vi "~sequence tester.vi"() -> ()   [LabVIEW 2017]
uses:
  Classes/Sequence/SequenceSubvis/TestStep.ctl
  Classes/Sequence/SequenceSubvis/RF Direction.ctl
  Classes/Sequence/SequenceSubvis/PolarizationSelect.ctl
  StepCmdProperties.ctl
  NewTestProperties.ctl
panel:
  out "New Setups":T1[](array[typedef])
  out "Array":T3[](array[typedef])
  in  "Sequence":T4[](array[typedef])
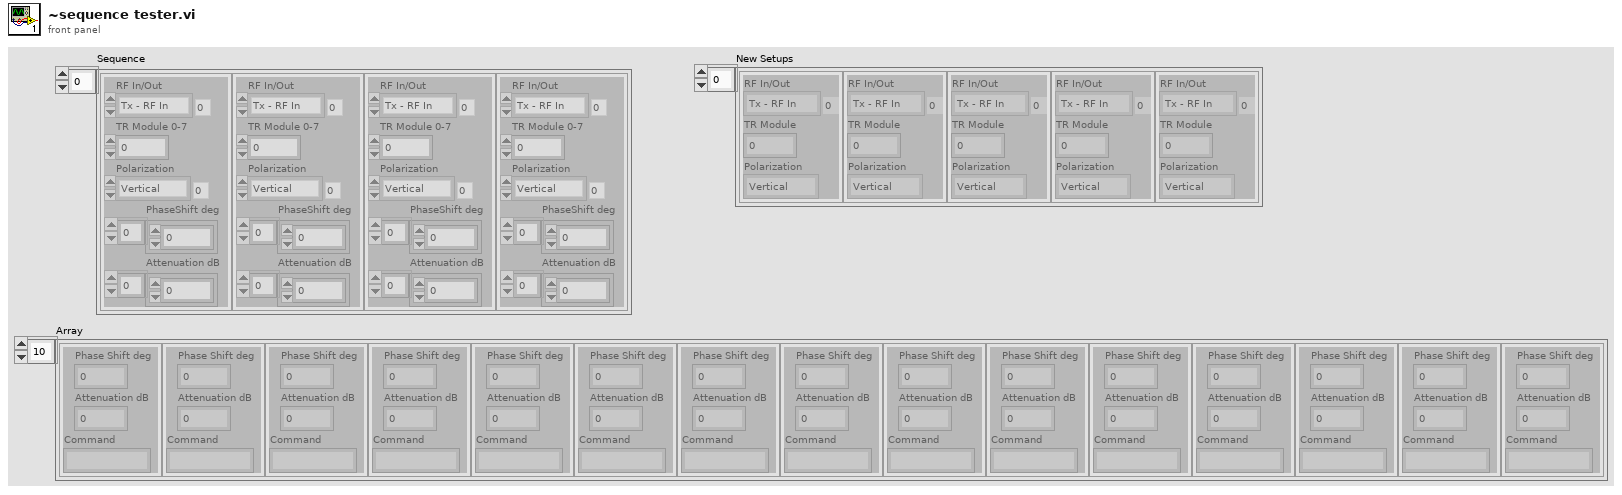
[diagram p1: front panel]
types:
  T1 = typedef "NewTestProperties.ctl" = cluster{"RF In/Out":T2, "TR Module":i32, "Polarization":enum16{"Vertical", "Horizontal"}}
  T2 = typedef "RF Direction.ctl" = enum16{"Tx - RF In", "Rx - RF Out"}
  T3 = typedef "StepCmdProperties.ctl" = cluster{"Phase Shift deg":dbl, "Attenuation dB":dbl, "Command":string}
  T4 = typedef "TestStep.ctl" = cluster{"RF In/Out":T2, "TR Module 0-7":i32, "Polarization":T5, "PhaseShift deg":dbl[], "Attenuation dB":dbl[]}
  T5 = typedef "PolarizationSelect.ctl" = enum16{"Vertical", "Horizontal"}
  T6 = cluster{"RF":enum16{"RF IN", "RF OUT"}, "TR Module":i32, "Polarization":enum16{"Vertical", "Horizontal"}}[]
  T7 = typedef "PatchNewTestStep.ctl" = cluster{"RF In/Out":T2, "TR Module":i32, "Polarization":T5}
  T8 = cluster{"RF In/Out":u16, "TR Module":i32, "Polarization":T5}[]
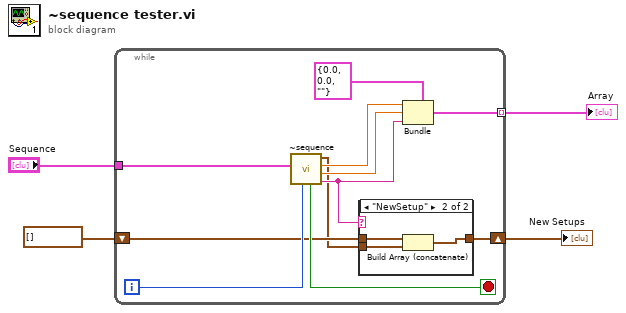
[diagram p0: block diagram]
diagram:
  n1 = while {
    tunnel: [w11] -> w4 mode=indexing
    tunnel: "Sequence" -> [w10]
    shift-right: [w6] -> w1
    shift-left: T6 [] -> [w8]
    i -> [w15]
    stop <- w14 stop-if-true
    n2 = call "~sequence.vi"("i"=w15, "Sequence"=w10) -> ("Command"=w9:string, "Attenuation dB"=w12:dbl, "Phase Shift deg"=w13:dbl, "NewSetup"=w7:T7, "Sequence is done"=w14:bool)  [unwired: 5 in]
    n3 = case shown="\"NewSetup\"" w9 {
      tunnel: w8 -> [w16 w19]
      tunnel: w7 -> [_ w18]
      tunnel: [w16 w17] -> w6
      frame "False", Default {
      }
      frame "NewSetup" {
        n4 = Build Array (concatenate)(w19, w18) -> (w17:T8)
      }
    }
    n5 = Bundle(cluster=T3 {"Phase Shift deg"=0.0, "Attenuation dB"=0.0, "Command"=""}, "Phase Shift deg"=w13, "Attenuation dB"=w12, "Command"=w9) -> (w11:T3)
  }
  "Array" <- w4
  "New Setups" <- w1
